vi "Read Error Code.vi"(8 "error in":errorcluster, 10 "Actuator Name":string, 11 "UTP IO Session in":T1) -> (0 "error out":errorcluster, 2 "Error Code":i16, 3 "UTP IO Session out":T1)   [LabVIEW 2023, in "Actuators.lvlib"]
doc: "Read Error Code and Error Text"
uses:
  Actuators.lvlib
  <vilib>/Noffz/UTP IO/UTP IO Library/Typedefs/Session Handle.ctl
  <vilib>/Noffz/UTP IO/UTP IO Library/UTP IO Pool Session.lvclass
  <vilib>/Noffz/UTP IO/UTP IO Library/methods/poly/plc/Read PLC Variable (I16).vi
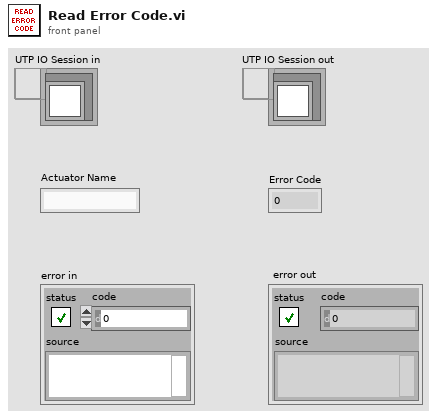
[diagram p1: front panel]
types:
  T1 = typedef "UTP IO Library.lvlib/UTP IO Pool Session.lvclass/Session Handle.ctl" = refnum<data-value>
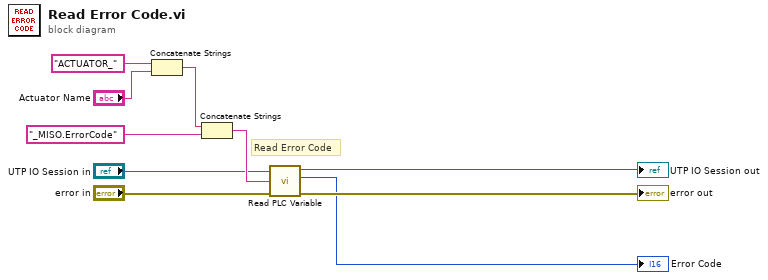
[diagram p0: block diagram]
diagram:
  # "Read Error Code"
  n1 = Concatenate Strings("ACTUATOR_" ("string"), "Actuator Name") -> (w2:string)
  n2 = Concatenate Strings(w2, "_MISO.ErrorCode" ("string")) -> (w10:string)
  n3 = call-poly <vilib>:"Read PLC Variable.vi"("error in (no error)"="error in", "variable name"=w10, "UTP IO Session in"="UTP IO Session in") -> ("error out"=→"error out":errorcluster, "value"=→"Error Code":i16, "UTP IO Session out"=→"UTP IO Session out":T1)  [unwired: 6 in]
